vi "Main.vi"() -> ()   [LabVIEW 2018]
uses:
  HV_QMH/HV QMH.lvlib
panel:
  in  "?":enum32{"Automated", "Monitor"}(tab)
  in  "Edit PMT File":bool
  in  "Off":bool
  in  "Apply":bool
  in  "PMT #":string[](array[string])
  in  "Channel":string[](array[string])
  in  "Test":string
  in  "Stop":bool
  out "?":T1
  # "In the final version, this section will contain extra controls for other hardware.\n\nIn this simplified automation demo, please enter up 12 PMT numbers and the channel they are connected to. Channels 0-5 are on board A and channels 6-11 are on\nboard B.\n\nThen select a test number. There are currently 4 tests; 1, 2, 3 and 4\n\nThe program will search the configuration file at HV_Automation_Demo/LabVIEW_Control/HV_Settings/HV_Settings.txt for the PMT and the voltaged at which to test at.\n\nThis can be edited by using the \"HV_Edit_PMT_File\" application. Press the \"Edit PMT File\" button to use this. Please read the \"Read Me\" section within this vi.\nNote: For this to work, the \"HV_Edit_PMT_File\" application must be built. Please see the read me files and how to build application files for further instruction.\n\nIf an invalid PMT number, channel or test is selected, the program will return a message saying so and will not turn channels on.\n\nOnce the values are entered (and the vi running if using the normal vi and not the application), press \"Apply\" to apply the settings and start the tests.\n\nUse the \"Monitor\" tab to monitor all values on the HV cards.\n\nTo turn the channels off, press the \"OFF\" button.\n\nPress the \"CLOSE\" button when finished to close the application or vi down. Pressing \"CLOSE\" will also ramp HV channels down."
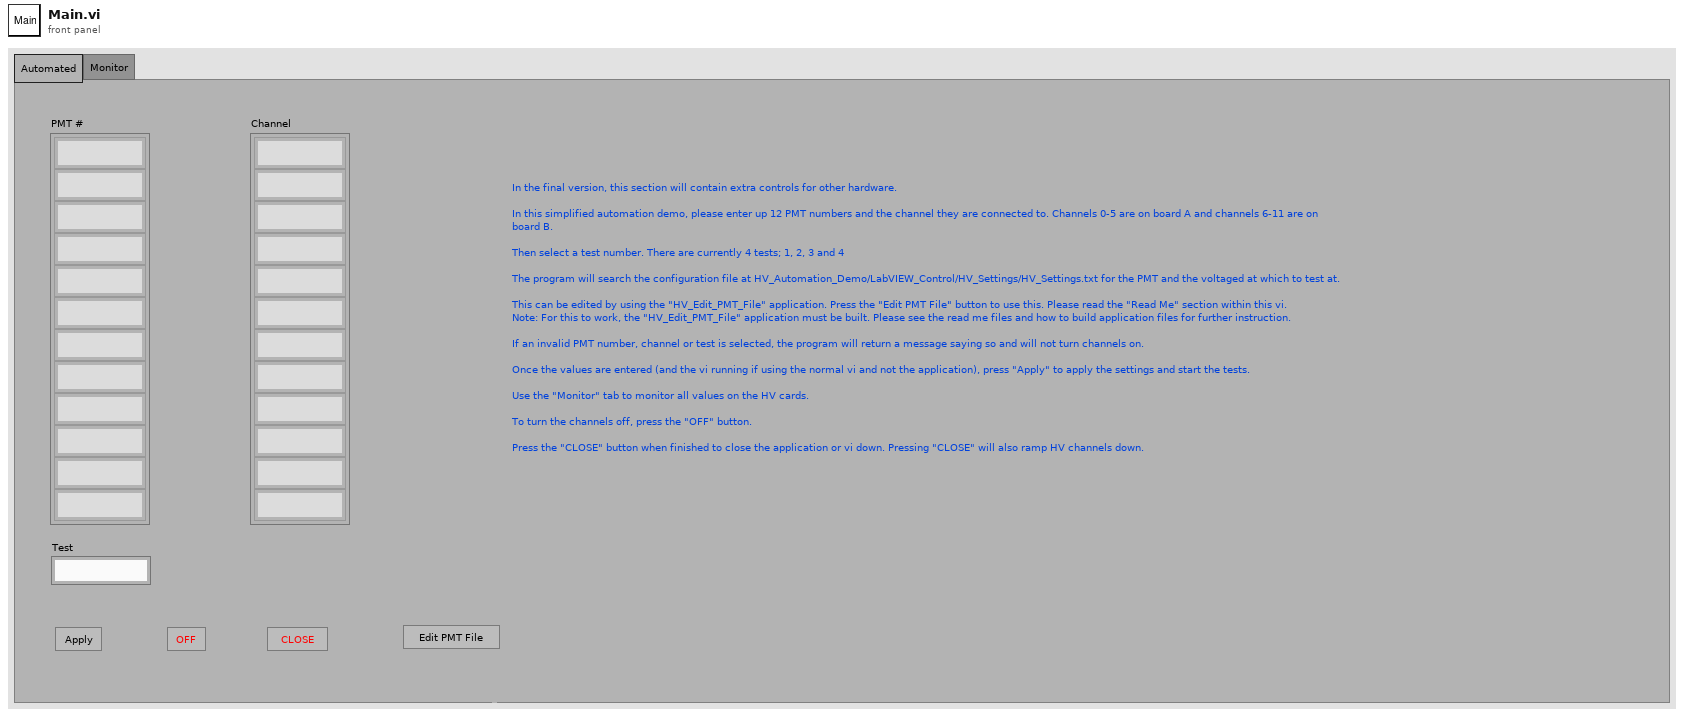
[diagram p1: front panel]
types:
  T1 = cluster{"Volt Monitor":string[][], "On/Off":bool[], "Rampup":bool[], "Rampdown":bool[], "Status Errors":string[], "Errors: (Err: 0 means no error)\nVolt monitor       Status":string[]}
  T2 = cluster{"Volt Monitor":string[][], "On/Off":bool[], "Rampup":bool[], "Rampdown":bool[], "Status Errors":string[], "Errors:\nVolt monitor                Status":string[]}
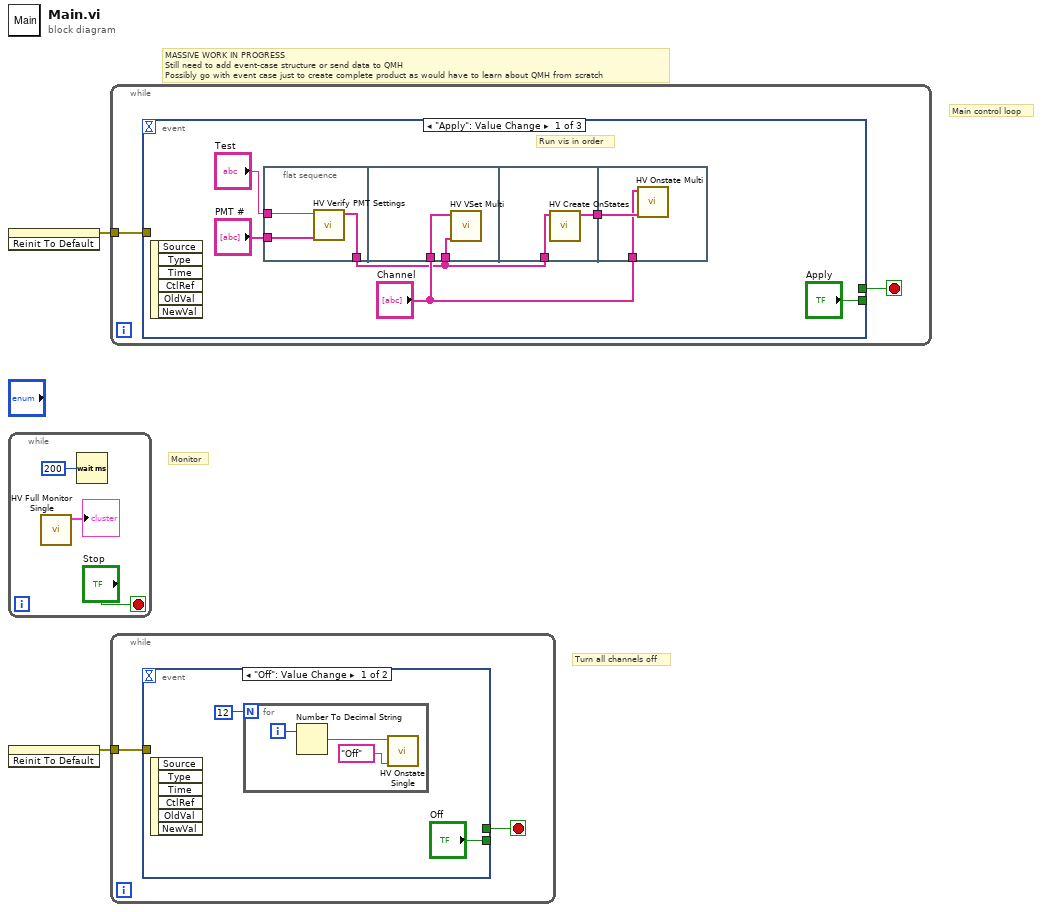
[diagram p0: block diagram]
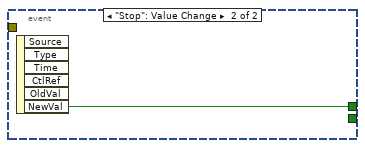
[diagram p2: hidden frame]
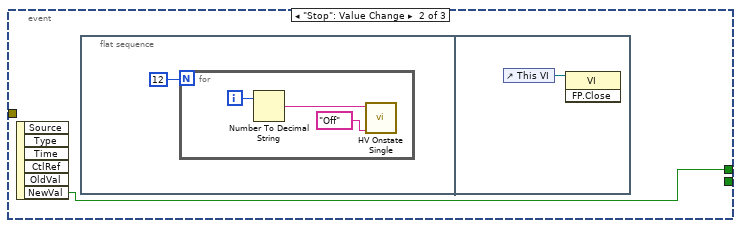
[diagram p3: hidden frame]
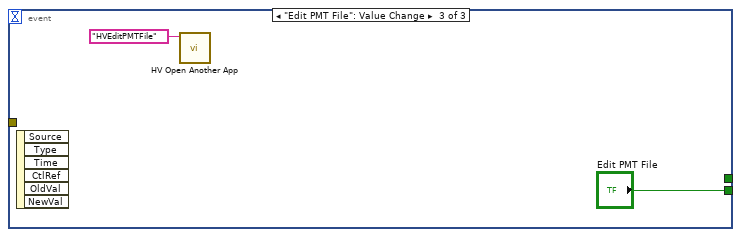
[diagram p4: hidden frame]
diagram:
  # "Monitor"
  # "Turn all channels off"
  # "Main control loop"
  # "MASSIVE WORK IN PROGRESS\nStill need to add event-case structure or send data to QMH\nPossibly go with event case just to create complete product as would have to learn about QMH from scratch"
  n1 = invoke on="Apply" class="Bool" method="Reinit To Default"() -> (error out=w2:errorcluster)  [unwired: 3 in, 2 out]
  n2 = while {
    stop <- "Stop" stop-if-true
    n3 = call "HV Full Monitor Single.vi"() -> ("Monitor Cluster"=→"?":T2)  [unwired: 11 in]
    n4 = Wait (ms)(milliseconds to wait=200) -> ()  [unwired: 1 out]
  }
  n5 = invoke on="Off" class="Bool" method="Reinit To Default"() -> (error out=w1:errorcluster)  [unwired: 3 in, 2 out]
  n6 = while {
    tunnel: w2 -> [w6]
    stop <- w7 stop-if-true
    n7 = event shown="[0] \"Apply\": Value Change" {
      selector: _ -> [_ _ _]
      dyn-events: _ -> [_ _ _]
      timeout: _ -> [_ _ _]
      tunnel: ["Apply" _ "Edit PMT File"] -> _
      tunnel: [_ w23 _] -> w7
      tunnel: w6 -> [_ _ _]
      event "Apply": Value Change {
        # "Run vis in order"
        n8 = event-data() -> ()  [unwired: 1 in, 6 out]
        n9 = flat-sequence {
          tunnel: "PMT #" -> [w16]
          tunnel: "Test" -> [w15]
          tunnel: [w14] -> w10
          tunnel: w10 -> [w18]
          tunnel: "Channel" -> [w17]
          tunnel: w10 -> [w20]
          tunnel: [w19] -> w12
          tunnel: w12 -> [w22]
          tunnel: "Channel" -> [w21]
          frame #0 {
            n10 = call "HV Verify PMT Settings.vi"("PMT's"=w16, "Test"=w15) -> ("Voltages"=w14:string[])  [unwired: 9 in]
          }
          frame #1 {
            n11 = call "HV VSet Multi.vi"("Voltage"=w18, "Channel"=w17) -> ()  [unwired: 9 in, 1 out]
          }
          frame #2 {
            n12 = call "HV Create OnStates.vi"("Voltages"=w20) -> ("Onstates"=w19:string[])  [unwired: 10 in]
          }
          frame #3 {
            n13 = call "HV Onstate Multi.vi"("On/Off"=w22, "Channel"=w21) -> ()  [unwired: 9 in, 1 out]
          }
        }
      }
      event "Stop": Value Change {
        n14 = event-data() -> ("NewVal"=w23:bool)  [unwired: 1 in, 5 out]
        n15 = flat-sequence {
          frame #0 {
            n16 = for {
              N: 12 -> [_]
              i -> [w27]
              n17 = Number To Decimal String(number=w27) -> (decimal integer string=w26:string)  [unwired: 1 in]
              n18 = call "HV Onstate Single.vi"("On/Off"="Off", "Channel"=w26) -> ()  [unwired: 9 in, 1 out]
            }
          }
          frame #1 {
            n19 = control-ref of="This VI"() -> (w28:refnum<vi>)
            n20 = invoke class="VI" method="FP.Close"(reference=w28) -> ()  [unwired: 2 in, 3 out]
          }
        }
      }
      event "Edit PMT File": Value Change {
        n21 = event-data() -> ()  [unwired: 1 in, 6 out]
        n22 = call "HV Open Another App.vi"("Vi Name"="HVEditPMTFile") -> ()  [unwired: 10 in, 1 out]
      }
    }
  }
  n23 = while {
    tunnel: w1 -> [w32]
    stop <- w31 stop-if-true
    n24 = event shown="[0] \"Off\": Value Change" {
      selector: _ -> [_ _]
      dyn-events: _ -> [_ _]
      timeout: _ -> [_ _]
      tunnel: ["Off" _] -> _
      tunnel: w32 -> [_ _]
      tunnel: [_ w38] -> w31
      event "Off": Value Change {
        n25 = event-data() -> ()  [unwired: 1 in, 6 out]
        n26 = for {
          N: 12 -> [_]
          i -> [w37]
          n27 = Number To Decimal String(number=w37) -> (decimal integer string=w36:string)  [unwired: 1 in]
          n28 = call "HV Onstate Single.vi"("On/Off"="Off", "Channel"=w36) -> ()  [unwired: 9 in, 1 out]
        }
      }
      event "Stop": Value Change {
        n29 = event-data() -> ("NewVal"=w38:bool)  [unwired: 1 in, 5 out]
      }
    }
  }
